vi "Generate File Test Case Table.vi"(8 "error in (no error)":errorcluster, 11 "LUnit Test Vector in":refnum<class "LUnit Test Vector.lvclass">) -> (0 "error out":errorcluster, 2 "Test Case Table":string, 3 "LUnit Test Vector out":refnum<class "LUnit Test Vector.lvclass">)   [LabVIEW 2020, in "LUnit Test Vector.lvclass"]
uses:
  LUnit Test Vector.lvclass
  LUnit Test Vector.lvclass/LUnit Test Vector.ctl
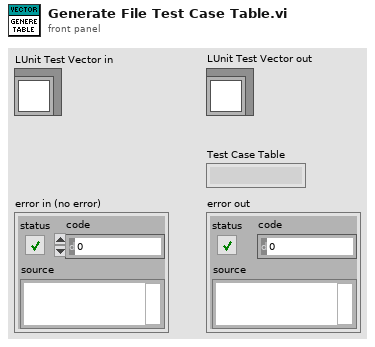
[diagram p1: front panel]
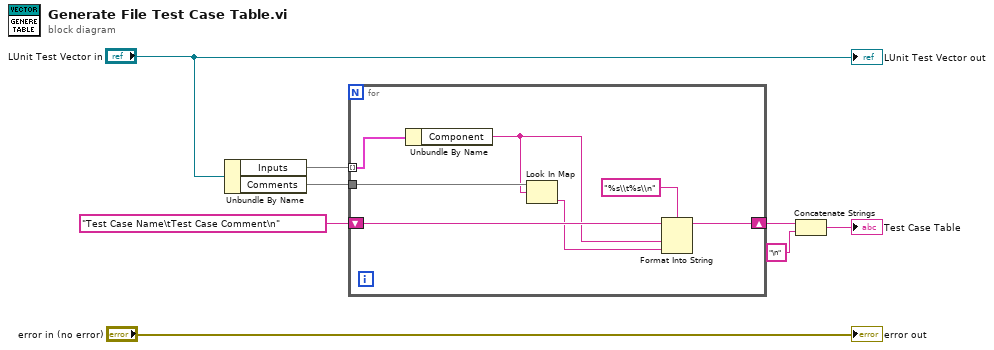
[diagram p0: block diagram]
diagram:
  n1 = Unbundle By Name("LUnit Test Vector in") -> ("Inputs"=w1:map{string, map{string, variant}}, "Comments"=w7:map{string, string})
  n2 = for {
    tunnel: w7 -> [w11]
    shift-right: [w13] -> w5
    shift-left: "Test Case Name\tTest Case Comment\n" -> [w14]
    tunnel: w1 -> [w12] mode=indexing
    n3 = Unbundle By Name(w12) -> ("Component"=w9:string)
    n4 = Look In Map(map=w11, key=w9) -> (value=w10:string)  [unwired: 1 in, 1 out]
    n5 = Format Into String(format string="%s\\t%s\\n", initial string=w14, w9, w10) -> (resulting string=w13:string)  [unwired: 1 in, 1 out]
  }
  n6 = Concatenate Strings(w5, "\n" ("string")) -> (→"Test Case Table":string)
  "error out" <- "error in (no error)"
  "LUnit Test Vector out" <- "LUnit Test Vector in"
